vi "MenuDo.vi"(0 "Column in":refnum<class "Column.lvclass">, 1 "Col Array Ref in":refnum<vi>, 2 "Layout Ring Refnum":refnum<vi>, 3 "Clipboard":refnum<vi>, 5 "ItemTag":string, 7 "VariableManagerRef":refnum<vi>, 9 "Table CtlRef In":refnum<vi>, 11 "error in (no error)":errorcluster, 12 "Cell Position":T1, 13 "ModeCol Index":i32=2, 14 "Table History ref":refnum<vi>) -> (4 "Column out":refnum<class "Column.lvclass">, 6 "Col Array Ref out":refnum<vi>, 8 "Update HWI?":bool, 10 "Table CtlRef Out":refnum<vi>, 15 "error out":errorcluster)   [LabVIEW 2013, in "Column.lvclass"]
doc: "Perform selected shortcut (right-click) menu actions for all columns in general.\nThis VI is read-only w.r.t column data."
uses:
  Column.lvclass
  <vilib>/Utility/miscctls.llb/LVRowAndColumnTypeDef.ctl
  TypeDefs/TableHistory.ctl
  TypeDefs/TableArray.ctl
  VariableManagerCodes/VariableManager/VariableManager.lvclass
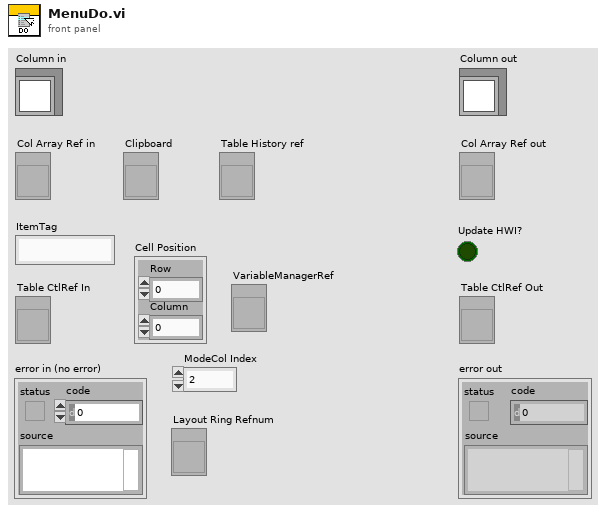
[diagram p1: front panel]
types:
  T1 = typedef "LVRowAndColumnTypeDef.ctl" = cluster{"Row":i32, "Column":i32}
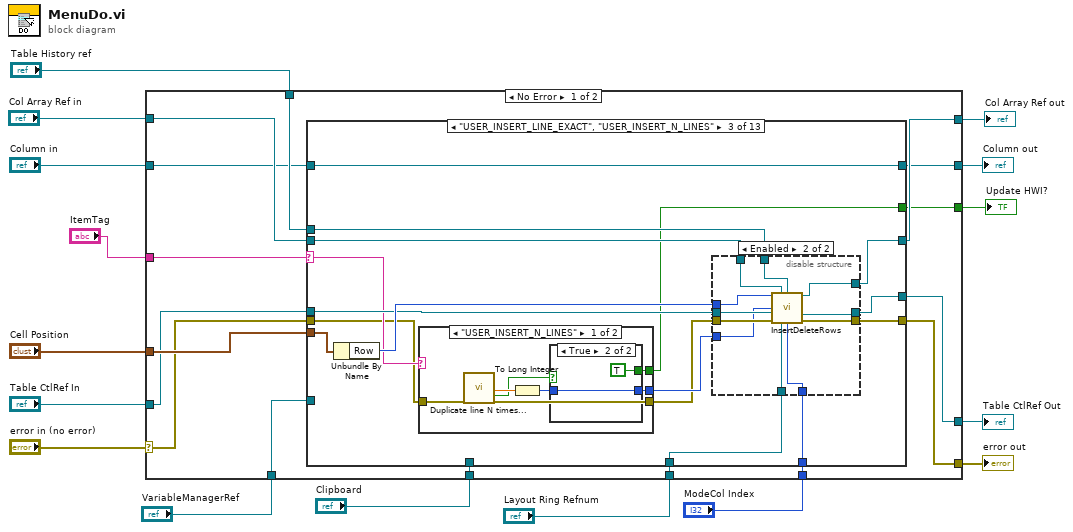
[diagram p0: block diagram]
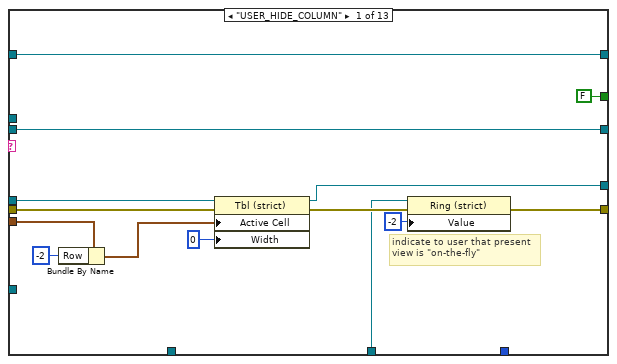
[diagram p2: hidden frame]
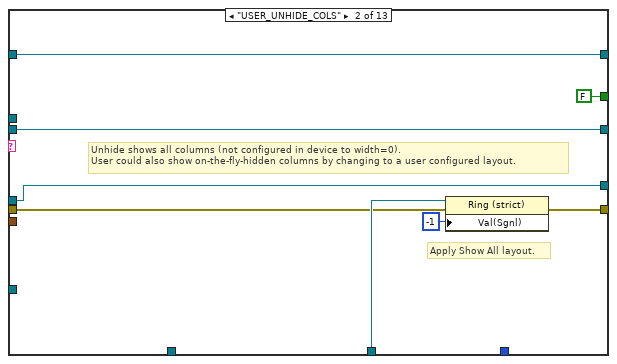
[diagram p3: hidden frame]
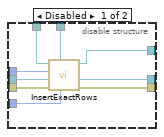
[diagram p4: hidden frame]
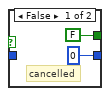
[diagram p5: hidden frame]
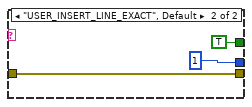
[diagram p6: hidden frame]
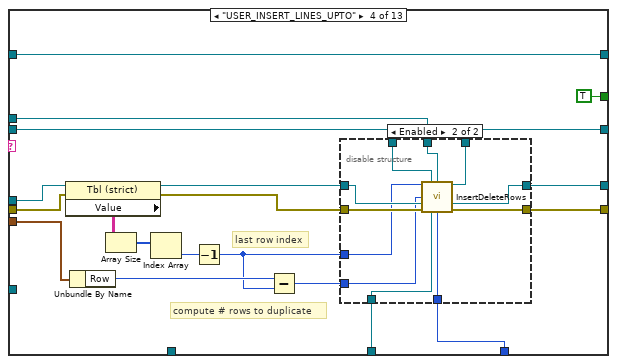
[diagram p7: hidden frame]
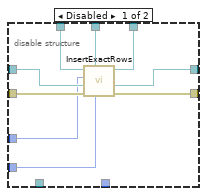
[diagram p8: hidden frame]
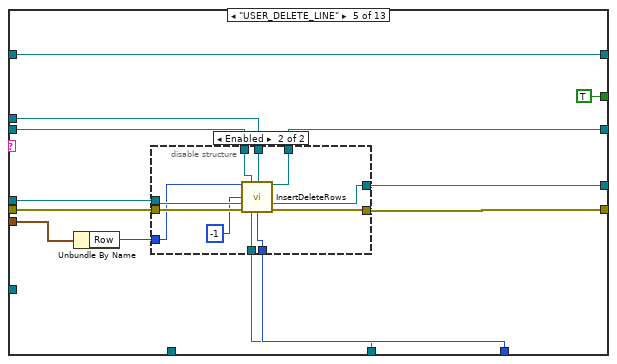
[diagram p9: hidden frame]
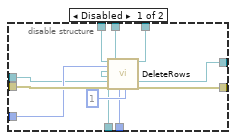
[diagram p10: hidden frame]
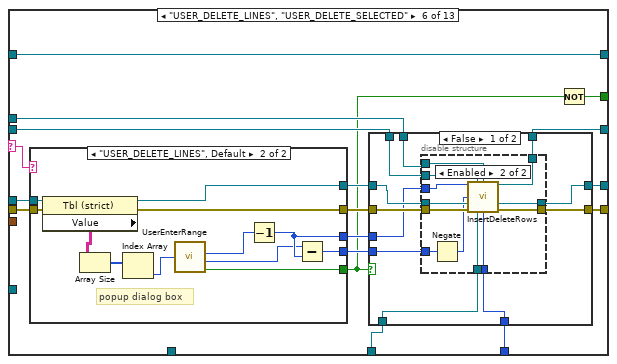
[diagram p11: hidden frame]
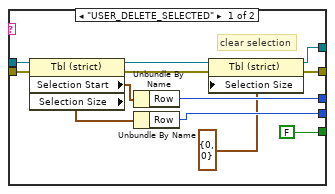
[diagram p12: hidden frame]
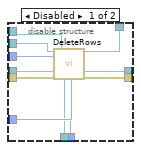
[diagram p13: hidden frame]
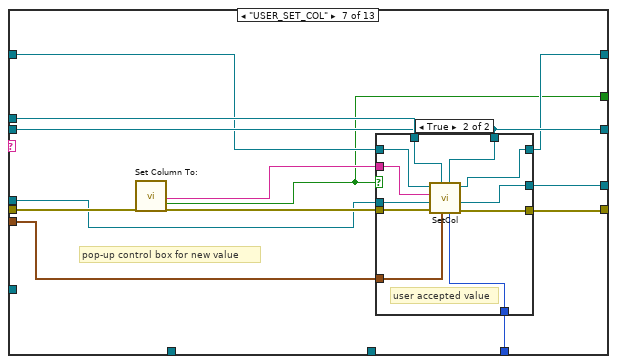
[diagram p15: hidden frame]
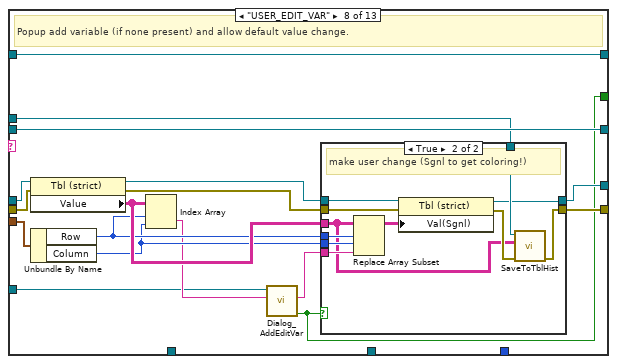
[diagram p17: hidden frame]
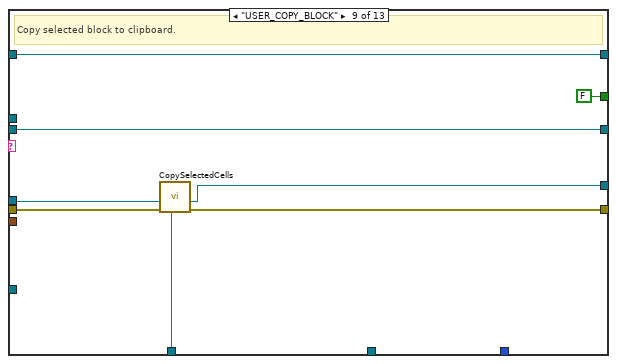
[diagram p19: hidden frame]
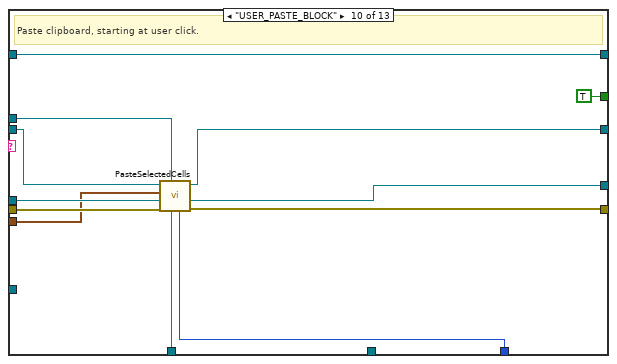
[diagram p20: hidden frame]
diagram:
  n1 = case shown="No Error" "error in (no error)" {
    selector: "error in (no error)" -> [w29 w371]
    tunnel: [w27 w371] -> w15
    tunnel: [w18 w370] -> w13
    tunnel: "Column in" -> [w19 w370]
    tunnel: "Table CtlRef In" -> [w30 w369]
    tunnel: [w28 w369] -> w11
    tunnel: "ItemTag" -> [w32 _]
    tunnel: "Cell Position" -> [w31 _]
    tunnel: [w25 w368] -> w7
    tunnel: "Col Array Ref in" -> [w26 w368]
    tunnel: "Clipboard" -> [w24 _]
    tunnel: "Table History ref" -> [w23 _]
    tunnel: "VariableManagerRef" -> [w22 _]
    tunnel: "ModeCol Index" -> [w21 _]
    tunnel: "Layout Ring Refnum" -> [w20 _]
    tunnel: [w17 FALSE ("Update HWI?")] -> w1
    frame No Error {
      n2 = case shown="\"USER_INSERT_LINE_EXACT\", \"USER_INSERT_N_LINES\"" w32 {
        selector: w32 -> [_ _ w64 _ _ w186 _ _ _ _ _ _ _]
        tunnel: w31 -> [w43 _ w70 w124 w157 _ w268 w298 _ w331 w337 _ _]
        tunnel: w30 -> [w45 w50 w67 w123 w154 w194 w264 w297 w319 w333 w341 w360 w366]
        tunnel: w29 -> [w46 w51 w63 w121 w156 w192 w265 w294 w321 w332 w343 w359 w365]
        tunnel: [w44 w50 w59 w109 w149 w196 w270 w300 w318 w330 w341 w346 w366] -> w28
        tunnel: [w37 w53 w58 w108 w148 w195 w269 w299 w320 w327 w342 w350 w365] -> w27
        tunnel: w26 -> [w39 w52 w68 w115 w153 w188 w262 w301 w322 w328 w339 w349 w364]
        tunnel: [w39 w52 w66 w114 w152 w187 w262 w301 w322 w329 w339 w347 w364] -> w25
        tunnel: w19 -> [w34 w48 w60 w110 w150 w184 w260 w286 w316 w324 w344 w361 w363]
        tunnel: w24 -> [_ _ _ _ _ _ _ _ w317 w334 _ _ _]
        tunnel: w23 -> [_ _ w61 w111 w151 w185 w263 w293 _ w326 w340 w348 _]
        tunnel: w22 -> [_ _ _ _ _ _ _ w287 _ _ w338 _ _]
        tunnel: w21 -> [_ _ w56 w107 w147 w183 w261 _ _ w325 w336 w351 _]
        tunnel: w20 -> [w36 w54 w57 w106 w146 w182 _ _ _ _ _ w352 _]
        tunnel: [w34 w48 w60 w110 w150 w184 w259 w286 w316 w324 w344 w361 w363] -> w18
        tunnel: [FALSE ("Update HWI?") FALSE ("Update HWI?") w55 TRUE ("Update HWI?") TRUE ("Update HWI?") w181 w258 w285 FALSE ("Update HWI?") TRUE ("Update HWI?") w335 TRUE ("Update HWI?") FALSE ("Update HWI?")] -> w17
        frame "USER_HIDE_COLUMN" {
          # "indicate to user that present\nview is \"on-the-fly\""
          n3 = Bundle By Name(cluster=w43, "Row"=-2) -> (w41:T1)
          n4 = property class="Tbl (strict)"(reference=w45, error in=w46, "Active Cell"=w41, "Width"=u32 0 ("Active Cell:Cell Size:Width")) -> (reference out=w44:refnum<vi>, error out=w38:errorcluster)
          n5 = property class="Ring (strict)"(reference=w36, error in=w38, "Value"=-2) -> (error out=w37:errorcluster)  [unwired: 1 out]
        }
        frame "USER_UNHIDE_COLS" {
          # "Unhide shows all columns (not configured in device to width=0).\nUser could also show on-the-fly-hidden columns by changing to a user configured layout."
          # "Apply Show All layout."
          n6 = property class="Ring (strict)"(reference=w54, error in=w51, "Val(Sgnl)"=-1 ("Value (Signaling)")) -> (error out=w53:errorcluster)  [unwired: 1 out]
        }
        frame "USER_INSERT_LINE_EXACT", "USER_INSERT_N_LINES" {
          n7 = Unbundle By Name(w70) -> ("Row"=w69:i32)
          n8 = case shown="\"USER_INSERT_N_LINES\"" w64 {
            tunnel: [w93 1 ("# rows")] -> w65
            tunnel: w63 -> [w96 w103]
            tunnel: [w95 w103] -> w62
            tunnel: [w91 TRUE ("Update HWI?")] -> w55
            frame "USER_INSERT_N_LINES" {
              n9 = call "Duplicate line N times..."("error in (no error)"=w96) -> ("Num lines"=w97:dbl, "OK"=w94:bool, "error out"=w95:errorcluster)  [unwired: 16 in]
              n10 = To Long Integer(number=w97) -> (32bit integer=w92:i32)
              n11 = case shown="True" w94 {
                tunnel: [0 w101] -> w93
                tunnel: w92 -> [_ w101]
                tunnel: [FALSE ("Update HWI?") TRUE ("Update HWI?")] -> w91
                frame False {
                  # "cancelled"
                }
                frame True {
                }
              }
            }
            frame "USER_INSERT_LINE_EXACT", Default {
            }
          }
          n12 = disable-structure shown="Enabled" {
            disable-tunnel: w69 -> [w79 w86]
            disable-tunnel: w68 -> [w78 w85]
            disable-tunnel: w67 -> [w77 w88]
            disable-tunnel: [w76 w83] -> w66
            disable-tunnel: w65 -> [w75 w82]
            disable-tunnel: w62 -> [w74 w90]
            disable-tunnel: w61 -> [w73 w84]
            disable-tunnel: [w72 w87] -> w59
            disable-tunnel: [w71 w89] -> w58
            disable-tunnel: w57 -> [_ w81]
            disable-tunnel: w56 -> [_ w80]
            frame Disabled {
              n13 = call "InsertExactRows.vi"("# rows"=w75, "Table History ref"=w73, "error in (no error)"=w74, "Table CtlRef In"=w77, "Row"=w79, "Col Array Ref in"=w78) -> ("error out"=w71:errorcluster, "Table CtlRef Out"=w72:refnum<vi>, "Col Array Ref out"=w76:refnum<vi>)  [unwired: 3 in]
            }
            frame Enabled {
              n14 = call "InsertDeleteRows.vi"("Start Row"=w86, "Col Array Ref in"=w85, "Table History ref"=w84, "# times (1)"=w82, "Table CtlRef In"=w88, "error in (no error)"=w90, "Layout Ring Refnum"=w81, "Mode Col Index"=w80) -> ("Col Array Ref out"=w83:refnum<vi>, "Table CtlRef Out"=w87:refnum<vi>, "error out"=w89:errorcluster)  [unwired: 5 in]
            }
          }
        }
        frame "USER_INSERT_LINES_UPTO" {
          # "last row index"
          # "compute # rows to duplicate"
          n15 = property class="Tbl (strict)"(reference=w123, error in=w121) -> (reference out=w122:refnum<vi>, error out=w120:errorcluster, "Value"=w119:string[][])
          n16 = Unbundle By Name(w124) -> ("Row"=w117:i32)
          n17 = Array Size(array=w119) -> (size(s)=w118:i32[])
          n18 = Index Array(array=w118) -> (element=w116:i32)  [unwired: 1 in]
          n19 = Decrement(x=w116) -> (x-1=w113:i32)
          n20 = Subtract(x=w117, y=w113) -> (x-y=w112:i32)
          n21 = disable-structure shown="Enabled" {
            disable-tunnel: w122 -> [w133 w142]
            disable-tunnel: w120 -> [w132 w144]
            disable-tunnel: w115 -> [w131 w138]
            disable-tunnel: [w130 w137] -> w114
            disable-tunnel: w113 -> [w129 w135]
            disable-tunnel: w112 -> [w128 w134]
            disable-tunnel: w111 -> [w127 w136]
            disable-tunnel: [w126 w141] -> w109
            disable-tunnel: [w125 w143] -> w108
            disable-tunnel: w107 -> [_ w140]
            disable-tunnel: w106 -> [_ w139]
            frame Disabled {
              n22 = call "InsertExactRows.vi"("# rows"=w128, "Table History ref"=w127, "error in (no error)"=w132, "Table CtlRef In"=w133, "Row"=w129, "Col Array Ref in"=w131) -> ("error out"=w125:errorcluster, "Table CtlRef Out"=w126:refnum<vi>, "Col Array Ref out"=w130:refnum<vi>)  [unwired: 3 in]
            }
            frame Enabled {
              n23 = call "InsertDeleteRows.vi"("Start Row"=w135, "Col Array Ref in"=w138, "Table History ref"=w136, "# times (1)"=w134, "Table CtlRef In"=w142, "error in (no error)"=w144, "Layout Ring Refnum"=w139, "Mode Col Index"=w140) -> ("Col Array Ref out"=w137:refnum<vi>, "Table CtlRef Out"=w141:refnum<vi>, "error out"=w143:errorcluster)  [unwired: 5 in]
            }
          }
        }
        frame "USER_DELETE_LINE" {
          n24 = Unbundle By Name(w157) -> ("Row"=w155:i32)
          n25 = disable-structure shown="Enabled" {
            disable-tunnel: w156 -> [w168 w179]
            disable-tunnel: w155 -> [w167 w169]
            disable-tunnel: w154 -> [w166 w173]
            disable-tunnel: w153 -> [w165 w174]
            disable-tunnel: [w164 w176] -> w152
            disable-tunnel: w151 -> [w162 w175]
            disable-tunnel: [w161 w177] -> w149
            disable-tunnel: [w160 w178] -> w148
            disable-tunnel: w147 -> [w159 w171]
            disable-tunnel: w146 -> [w158 w172]
            frame Disabled {
              n26 = call "DeleteRows.vi"("Col Array Ref in"=w165, "Start Row"=w167, "Layout Ring Refnum"=w158, "Mode Col Index"=w159, "Table CtlRef In"=w166, "error in (no error)"=w168, "Table History ref"=w162, "# rows"=1) -> ("Col Array Ref out"=w164:refnum<vi>, "Table CtlRef Out"=w161:refnum<vi>, "error out"=w160:errorcluster)  [unwired: 9 in]
            }
            frame Enabled {
              n27 = call "InsertDeleteRows.vi"("Start Row"=w169, "Col Array Ref in"=w174, "Table History ref"=w175, "# times (1)"=-1, "Table CtlRef In"=w173, "error in (no error)"=w179, "Layout Ring Refnum"=w172, "Mode Col Index"=w171) -> ("Col Array Ref out"=w176:refnum<vi>, "Table CtlRef Out"=w177:refnum<vi>, "error out"=w178:errorcluster)  [unwired: 5 in]
            }
          }
        }
        frame "USER_DELETE_LINES", "USER_DELETE_SELECTED" {
          n28 = case shown="\"USER_DELETE_LINES\", Default" w186 {
            tunnel: w194 -> [w208 w220]
            tunnel: [w199 w219] -> w193
            tunnel: w192 -> [w207 w218]
            tunnel: [w198 w217] -> w191
            tunnel: [FALSE ("Canceled?") w213] -> w180
            tunnel: [w203 w210] -> w190
            tunnel: [w202 w211] -> w189
            frame "USER_DELETE_SELECTED" {
              # "clear selection"
              n29 = property class="Tbl (strict)"(reference=w208, error in=w207) -> (reference out=w200:refnum<vi>, error out=w201:errorcluster, "Selection Start"=w205:T1, "Selection Size"=w204:T1)
              n30 = Unbundle By Name(w205) -> ("Row"=w203:i32)
              n31 = Unbundle By Name(w204) -> ("Row"=w202:i32)
              n32 = property class="Tbl (strict)"(reference=w200, error in=w201, "Selection Size"=T1 {"Row"=0, "Column"=0} ("Selection Start")) -> (reference out=w199:refnum<vi>, error out=w198:errorcluster)
            }
            frame "USER_DELETE_LINES", Default {
              # "popup dialog box"
              n33 = property class="Tbl (strict)"(reference=w220, error in=w218) -> (reference out=w219:refnum<vi>, error out=w217:errorcluster, "Value"=w216:string[][])
              n34 = Array Size(array=w216) -> (size(s)=w215:i32[])
              n35 = Index Array(array=w215) -> (element=w214:i32)  [unwired: 1 in]
              n36 = call "UserEnterRange.vi"("Max Entry"=w214) -> ("Begin Out"=w212:i32, "End Out"=w209:i32, "Canceled?"=w213:bool)  [unwired: 1 in]
              n37 = Decrement(x=w212) -> (x-1=w210:i32)
              n38 = Subtract(x=w209, y=w210) -> (x-y=w211:i32)
            }
          }
          n39 = case shown="False" w180 {
            tunnel: [w224 w257] -> w196
            tunnel: [w223 w256] -> w195
            tunnel: w193 -> [w231 w257]
            tunnel: w191 -> [w230 w256]
            tunnel: w190 -> [w227 _]
            tunnel: w189 -> [w226 _]
            tunnel: w188 -> [w229 w255]
            tunnel: [w228 w255] -> w187
            tunnel: w185 -> [w225 _]
            tunnel: w183 -> [w222 _]
            tunnel: w182 -> [w221 _]
            frame False {
              n40 = disable-structure shown="Enabled" {
                disable-tunnel: w231 -> [w242 w250]
                disable-tunnel: w230 -> [w241 w253]
                disable-tunnel: w229 -> [w240 w247]
                disable-tunnel: [w239 w248] -> w228
                disable-tunnel: w227 -> [w238 w245]
                disable-tunnel: w226 -> [w237 w244]
                disable-tunnel: w225 -> [w236 w246]
                disable-tunnel: [w235 w249] -> w224
                disable-tunnel: [w234 w254] -> w223
                disable-tunnel: w222 -> [w233 w252]
                disable-tunnel: w221 -> [w232 w251]
                frame Disabled {
                  n41 = call "DeleteRows.vi"("Col Array Ref in"=w240, "Start Row"=w238, "Layout Ring Refnum"=w232, "Mode Col Index"=w233, "Table CtlRef In"=w242, "error in (no error)"=w241, "Table History ref"=w236, "# rows"=w237) -> ("Col Array Ref out"=w239:refnum<vi>, "Table CtlRef Out"=w235:refnum<vi>, "error out"=w234:errorcluster)  [unwired: 9 in]
                }
                frame Enabled {
                  n42 = Negate(x=w244) -> (-x=w243:i32)
                  n43 = call "InsertDeleteRows.vi"("Start Row"=w245, "Col Array Ref in"=w247, "Table History ref"=w246, "# times (1)"=w243, "Table CtlRef In"=w250, "error in (no error)"=w253, "Layout Ring Refnum"=w251, "Mode Col Index"=w252) -> ("Col Array Ref out"=w248:refnum<vi>, "Table CtlRef Out"=w249:refnum<vi>, "error out"=w254:errorcluster)  [unwired: 5 in]
                }
              }
            }
            frame True {
              # "user cancelled"
            }
          }
          n44 = Not(x=w180) -> (.not. x?=w181:bool)
        }
        frame "USER_SET_COL" {
          # "pop-up control box for new value"
          n45 = call "Set Column To:"("error in (no error)"=w265) -> ("value"=w267:string, "OK"=w258:bool, "error out"=w266:errorcluster)  [unwired: 16 in]
          n46 = case shown="True" w258 {
            tunnel: w266 -> [w273 w284]
            tunnel: [w272 w283] -> w270
            tunnel: [w273 w282] -> w269
            tunnel: w268 -> [_ w281]
            tunnel: w267 -> [_ w280]
            tunnel: w260 -> [w271 w279]
            tunnel: w264 -> [w272 w278]
            tunnel: w263 -> [_ w277]
            tunnel: w262 -> [_ w276]
            tunnel: w261 -> [_ w275]
            tunnel: [w271 w274] -> w259
            frame False {
              # "user cancelled"
            }
            frame True {
              # "user accepted value"
              n47 = call-dynamic "SetCol.vi"("ModeCol Index"=w275, "Col Array Ref in"=w276, "Cell Position"=w281, "Table History ref"=w277, "error in (no error)"=w284, "Table CtlRef In"=w278, "SetTo"=w280, "Column in"=w279) -> ("error out"=w282:errorcluster, "Table CtlRef Out"=w283:refnum<vi>, "Column out"=w274:refnum<class "Column.lvclass">)  [unwired: 1 out]
            }
          }
        }
        frame "USER_EDIT_VAR" {
          # "Popup add variable (if none present) and allow default value change."
          n48 = property class="Tbl (strict)"(reference=w297, error in=w294) -> (reference out=w296:refnum<vi>, error out=w295:errorcluster, "Value"=w292:string[][])
          n49 = Unbundle By Name(w298) -> ("Row"=w291:i32, "Column"=w290:i32)
          n50 = Index Array(array=w292, index (row)=w291, index (col)=w290) -> (element=w288:string)
          n51 = call "Dialog_AddEditVar.vi"("String in"=w288, "VariableManagerRef"=w287) -> ("OK?"=w285:bool, "Variable Name"=w289:string)  [unwired: 8 in]
          n52 = case shown="True" w285 {
            tunnel: w296 -> [w303 w312]
            tunnel: [w303 w311] -> w300
            tunnel: w295 -> [w302 w310]
            tunnel: [w302 w313] -> w299
            tunnel: w291 -> [_ w307]
            tunnel: w290 -> [_ w306]
            tunnel: w289 -> [_ w305]
            tunnel: w293 -> [_ w314]
            tunnel: w292 -> [_ w304]
            frame False {
              # "user cancelled"
            }
            frame True {
              # "make user change (Sgnl to get coloring!)"
              n53 = Replace Array Subset(array=w304, new element=w305, index (row)=w307, index (col)=w306) -> (w308:string[][])
              n54 = property class="Tbl (strict)"(reference=w312, error in=w310, "Val(Sgnl)"=w308) -> (reference out=w311:refnum<vi>, error out=w309:errorcluster)
              n55 = call "SaveToTblHist.vi"("error in (no error)"=w309, "OldTable (reset)"=w304, "Table History ref"=w314) -> ("error out"=w313:errorcluster)  [unwired: 8 in]
            }
          }
        }
        frame "USER_COPY_BLOCK" {
          # "Copy selected block to clipboard."
          n56 = call "CopySelectedCells.vi"("Clipboard"=w317, "error in (no error)"=w321, "Table CtlRef In"=w319) -> ("error out"=w320:errorcluster, "Table CtlRef Out"=w318:refnum<vi>)  [unwired: 7 in]
        }
        frame "USER_PASTE_BLOCK" {
          # "Paste clipboard, starting at user click."
          n57 = call "PasteSelectedCells.vi"("ModeCol Index"=w325, "Clipboard"=w334, "Table History ref"=w326, "error in (no error)"=w332, "Table CtlRef In"=w333, "Cell Start"=w331, "Col Array Ref in"=w328) -> ("error out"=w327:errorcluster, "Table CtlRef Out"=w330:refnum<vi>, "Col Array Ref out"=w329:refnum<vi>)  [unwired: 2 in]
        }
        frame "USER_SET_BLOCK" {
          # "Prompt user to choose value/variable and change entire block to that value"
          n58 = call "Dialog_SetBlockTo.vi"("ModeCol Index"=w336, "Cell Position"=w337, "Table History ref"=w340, "error in (no error)"=w343, "Table CtlRef In"=w341, "VariableManagerRef"=w338, "Col Array Ref in"=w339) -> ("error out"=w342:errorcluster, "OK"=w335:bool)  [unwired: 3 in]
        }
        frame "USER_DUPLICATE_SELECTED" {
          # "Called with N-row-wise selection: insert N lines after selection and paste selected cells there"
          n59 = property class="Tbl (strict)"(reference=w360, error in=w359) -> (reference out=w355:refnum<vi>, error out=w353:errorcluster, "Selection Start"=w358:T1, "Selection Size"=w357:T1)
          n60 = Unbundle By Name(w358) -> ("Row"=w356:i32)
          n61 = Unbundle By Name(w357) -> ("Row"=w354:i32)
          n62 = call "InsertDeleteRows.vi"("Start Row"=w356, "Col Array Ref in"=w349, "Table History ref"=w348, "sel size (1)"=w354, "Table CtlRef In"=w355, "error in (no error)"=w353, "Layout Ring Refnum"=w352, "Mode Col Index"=w351) -> ("Col Array Ref out"=w347:refnum<vi>, "Table CtlRef Out"=w346:refnum<vi>, "error out"=w350:errorcluster)  [unwired: 5 in]
        }
        frame Default {
        }
      }
    }
    frame Error {
    }
  }
  "error out" <- w15
  "Column out" <- w13
  "Table CtlRef Out" <- w11
  "Col Array Ref out" <- w7
  "Update HWI?" <- w1
